vi "UI_Show_Hide_Controls.vi"(8 "error in (no error)":errorcluster, 10 "Enable ?":bool, 11 "Controls":refnum<vi>[](array[refnum])) -> (0 "error out":errorcluster caption="sortie d'erreur")   [LabVIEW 2018]
doc: "Définit toutes les commandes du tableau en entrée à la valeur \"État Activé\"."
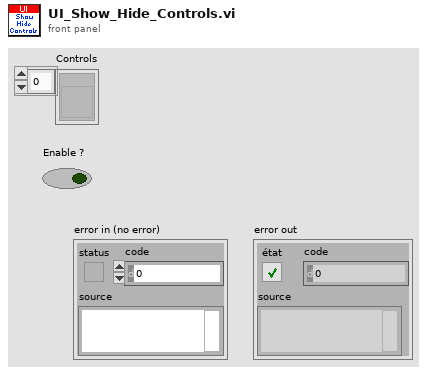
[diagram p1: front panel]
types:
  T1 = enum8{"Enabled", "Disabled", "Disabled and Grayed Out"}
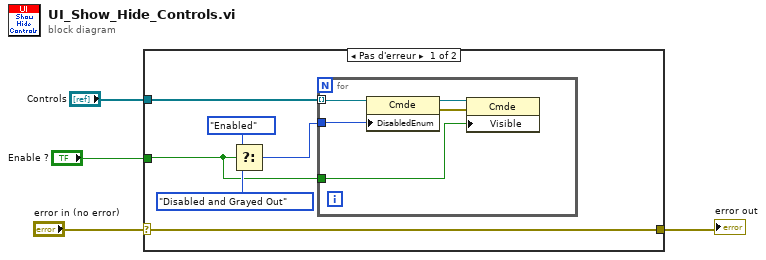
[diagram p0: block diagram]
diagram:
  n1 = case shown="Pas d'erreur" "error in (no error)" {
    selector: "error in (no error)" -> [w6 w16]
    tunnel: "Controls" -> [w10 _]
    tunnel: "Enable ?" -> [w5 _]
    tunnel: [w6 w16] -> w1
    frame No Error {
      n2 = Select(t=T1."Enabled" ("Désactivé"), s=w5, f=T1."Disabled and Grayed Out" ("Désactivé")) -> (s? t:f=w9:T1)
      n3 = for {
        tunnel: w10 -> [w15] mode=indexing
        tunnel: w9 -> [w14]
        tunnel: w5 -> [w11]
        n4 = property class="Cmde"(reference=w15, "DisabledEnum"=w14) -> (reference out=w13:refnum<vi>, error out=w12:errorcluster)  [unwired: 1 in]
        n5 = property class="Cmde"(reference=w13, error in=w12, "Visible"=w11) -> ()  [unwired: 2 out]
      }
    }
    frame Error {
    }
  }
  "error out" <- w1
